vi "retrieveMotionProfile.vi"() -> (0 "rightTraj":dbl[][](array[numeric]), 2 "leftTraj":dbl[][](array[numeric]))   [LabVIEW 2017]
uses:
  <vilib>/Rock Robotics/Network Tables/NT Read Numeric Array.vi
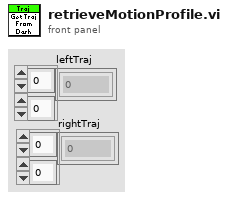
[diagram p1: front panel]
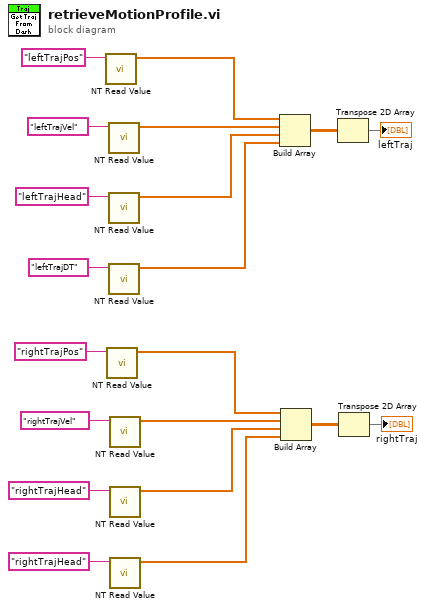
[diagram p0: block diagram]
diagram:
  n1 = call-poly <vilib>:"NT Read Value.vi"("Name"="leftTrajPos") -> ("Numeric Array"=w16:dbl[])  [unwired: 9 in, 1 out]
  n2 = call-poly <vilib>:"NT Read Value.vi"("Name"="rightTrajPos") -> ("Numeric Array"=w6:dbl[])  [unwired: 9 in, 1 out]
  n3 = call-poly <vilib>:"NT Read Value.vi"("Name"="leftTrajVel") -> ("Numeric Array"=w15:dbl[])  [unwired: 9 in, 1 out]
  n4 = call-poly <vilib>:"NT Read Value.vi"("Name"="leftTrajHead") -> ("Numeric Array"=w14:dbl[])  [unwired: 9 in, 1 out]
  n5 = call-poly <vilib>:"NT Read Value.vi"("Name"="leftTrajDT") -> ("Numeric Array"=w13:dbl[])  [unwired: 9 in, 1 out]
  n6 = call-poly <vilib>:"NT Read Value.vi"("Name"="rightTrajVel") -> ("Numeric Array"=w5:dbl[])  [unwired: 9 in, 1 out]
  n7 = call-poly <vilib>:"NT Read Value.vi"("Name"="rightTrajHead") -> ("Numeric Array"=w4:dbl[])  [unwired: 9 in, 1 out]
  n8 = call-poly <vilib>:"NT Read Value.vi"("Name"="rightTrajHead") -> ("Numeric Array"=w3:dbl[])  [unwired: 9 in, 1 out]
  n9 = Build Array(w16, w15, w14, w13) -> (w12:dbl[][])
  n10 = Build Array(w6, w5, w4, w3) -> (w2:dbl[][])
  n11 = Transpose 2D Array(2D array=w12) -> (transposed array=→"leftTraj":dbl[][])
  n12 = Transpose 2D Array(2D array=w2) -> (transposed array=→"rightTraj":dbl[][])
